vi "Get QObject LVClass.vi"(11 "LVLib":refnum<vi>) -> (2 "QObject":refnum<vi>, 3 "LVLib Dup":refnum<vi>)   [LabVIEW 2013]
panel:
  out "DEBUG Class Name":string
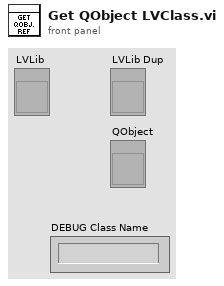
[diagram p1: front panel]
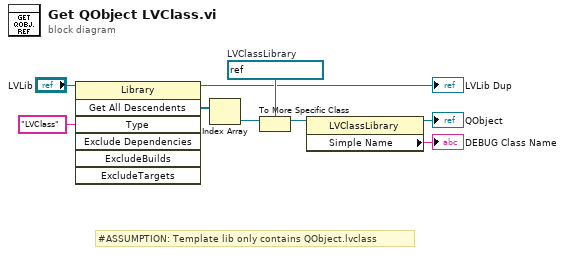
[diagram p0: block diagram]
diagram:
  w8 = refnum<vi> refnum  # LVClassLibrary
  # "#ASSUMPTION: Template lib only contains QObject.lvclass"
  n1 = invoke class="Library" method="Get All Descendents"(reference="LVLib", "Type"="LVClass") -> (reference out=→"LVLib Dup":refnum<vi>, "All Descendents"=w7:refnum<vi>[])  [unwired: 5 in, 5 out]
  n2 = Index Array(array=w7) -> (element=w6:refnum<vi>)  [unwired: 1 in]
  n3 = To More Specific Class(target class=w8, reference=w6) -> (specific class reference=w5:refnum<vi>)  [unwired: 1 in, 1 out]
  n4 = property class="LVClassLibrary"(reference=w5) -> (reference out=→"QObject":refnum<vi>, "Simple Name"=→"DEBUG Class Name":string)  [unwired: 1 in, 1 out]
